vi "PolhemusDataCollect.vi"(0 "Data Queue":refnum<queue>, 1 "Timed Structure Name":string, 2 "Timing Source":string="1 kHz", 5 "VISA resource name":refnum<visa-resource-name>, 7 "Bytes to Read":i32, 9 "Relative Time":u32, 11 "error in (no error)":errorcluster, 12 "Timed Loop Priority":i32=100, 13 "Time Bytes Before Output":i32, 14 "Sync In? (F)":bool) -> (4 "Queue Out":refnum<queue>, 6 "VISA resource name out":refnum<visa-resource-name>, 8 "Timing Array":u32[](array[numeric]), 15 "error out":errorcluster)   [LabVIEW 2009]
doc: "Collects data from the Polhemus Fastrak.\nUsing the number of bytes in the output of the polhemus, this program reads data from the serial port and sends it to a queue. Additionally, using the Relative Time command and the Time Bytes Before Output, this program will send a timestamp (in ms) with the output in the given number of bytes."
uses:
  <vilib>/Platform/TimedLoop/XDataNode/XDataNode.xnode
  <vilib>/Platform/TimedLoop/XDataNode/loadlvalarms.vi
  <vilib>/Platform/TimedLoop/XDataNode/timing_clust.ctl
  <vilib>/Platform/TimedLoop/XDataNode/nitl_modes.ctl
  <vilib>/Platform/TimedLoop/XDataNode/wakeup.ctl
  GlobalVariables.vi
  <vilib>/Platform/TimedLoop/XDataNode/XDNodeRunTimeDep.lvlib
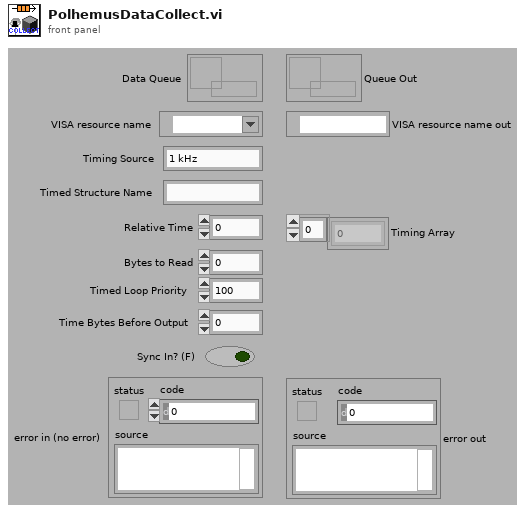
[diagram p1: front panel]
types:
  T1 = typedef "XDNodeRunTimeDep.lvlib/timing_clust.ctl" = cluster{"Expected End [f-1]":u64, "Actual End [f-1]":u64, "Finished Late? [f-1]":bool, "Expected End [i-1]":u64, "Actual End [i-1]":u64, "Finished Late? [i-1]":bool, "Expected Start [i]":u64, "Actual Start [i]":u64, "Expected Start [f]":u64, "Actual Start [f]":u64, "Source Name":string, "Structure Name":string, "Period":i64, "Deadline":i64, "Offset":i64, "Start":i64, "Priority":i32, "Timeout":i32, "Mode":T2, "Wakeup Reason":T3, "Error":errorcluster, "Source Type":string, "Secondary Source Type":string, "Global End Time":u64, "Global Start Time":u64, "Frame Duration":u64, "Iteration Duration":u64, "Assigned CPU":i32, "I/O Scan Engine Mode":u32}
  T2 = typedef "XDNodeRunTimeDep.lvlib/nitl_modes.ctl" = enum32{"No Change", "Process missed periods, maintain original phase", "Discard missed periods, maintain original phase", "Process missed periods, ignore original phase", "Discard missed periods, ignore original phase"}
  T3 = typedef "XDNodeRunTimeDep.lvlib/wakeup.ctl" = enum32{"Normal", "Aborted", "Asynchronous wakeup", "Timing source error", "Timed loop error", "Timeout"}
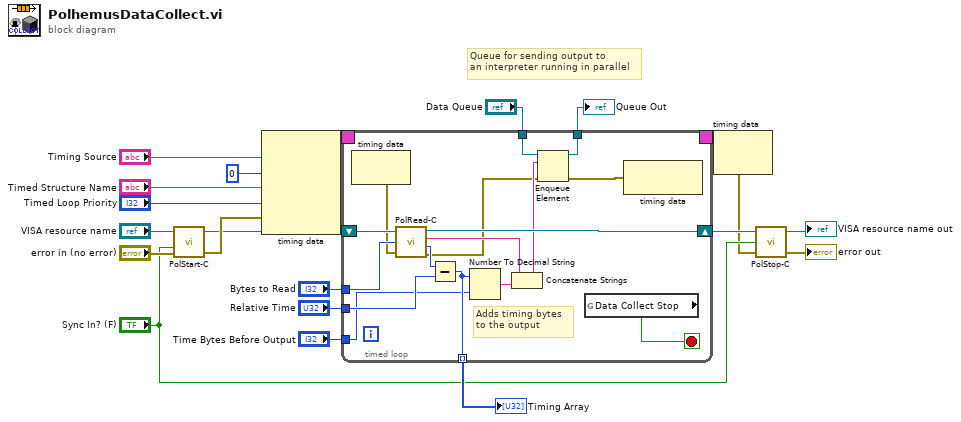
[diagram p0: block diagram]
diagram:
  # "Queue for sending output to\nan interpreter running in parallel"
  n1 = call "PolStart-C.vi"("error in (no error)"="error in (no error)", "Sync In? (F)"="Sync In? (F)", "VISA resource name"="VISA resource name") -> ("error out"=w7:errorcluster, "VISA resource name out"=w6:refnum<visa-resource-name>)  [unwired: 1 in]
  n2 = node-c288("Timing Source", i64 0 ("Period"), "Timed Structure Name", "Timed Loop Priority", w7) -> (w21:T1)
  n3 = timed-loop {
    timing: w21 -> [_]
    timing-out: [_] -> w20
    tunnel: "Bytes to Read" -> [w36]
    shift-right: [w35] -> w10
    shift-left: w6 -> [w37]
    tunnel: "Data Queue" -> [w34]
    tunnel: [w33] -> w11
    tunnel: "Relative Time" -> [w29]
    tunnel: [w26] -> w4 mode=indexing
    tunnel: "Time Bytes Before Output" -> [w25]
    stop <- w24 stop-if-true
    # "Adds timing bytes\nto the output"
    n4 = node-c288() -> (w32:errorcluster)  [unwired: 1 in]
    n5 = call "PolRead-C.vi"("VISA resource name"=w37, "Byte Sum"=w36, "error in (no error)"=w32) -> ("VISA resource name out"=w35:refnum<visa-resource-name>, "Polhemus Output"=w28:string, "Time"=w30:u32, "error out"=w23:errorcluster)
    n6 = Subtract(x=w30, y=w29) -> (x-y=w26:u32)
    n7 = Number To Decimal String(number=w26, width (-)=w25) -> (decimal integer string=w31:string)
    n8 = Concatenate Strings(w31, w28) -> (w27:string)
    n9 = Enqueue Element(queue=w34, element=w27, error in (no error)=w23) -> (queue out=w33:refnum<queue>, error out=w22:errorcluster)  [unwired: 1 in, 1 out]
    n10 = global read "GlobalVariables.vi" "Data Collect Stop"() -> (w24:bool)
    n11 = node-c288(w22) -> ()  [unwired: 1 out]
  }
  "Queue Out" <- w11
  "Timing Array" <- w4
  n12 = node-c288(w20) -> (w1:errorcluster)
  n13 = call "PolStop-C.vi"("error in (no error)"=w1, "Sync In? (F)"="Sync In? (F)", "VISA resource name"=w10) -> ("error out"=→"error out":errorcluster, "VISA resource name out"=→"VISA resource name out":refnum<visa-resource-name>)  [unwired: 1 in]
